vi "OpenVIFile.vi"(7 "error in (no error)":errorcluster, 8 "Pdf file path":path) -> (1 "error out":errorcluster)   [LabVIEW 2015]
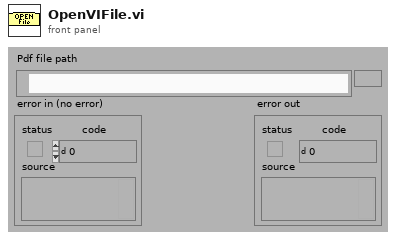
[diagram p1: front panel]
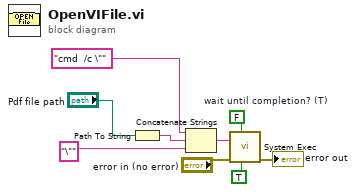
[diagram p0: block diagram]
diagram:
  w9 = FALSE  # wait until completion? (T)
  n1 = Path To String(path="Pdf file path") -> (string=w4:string)
  n2 = Concatenate Strings("cmd  /c \"", w4, "\"") -> (w6:string)
  n3 = call <vilib>:"System Exec.vi"("run minimized? (F)"=TRUE, "wait until completion? (T)"=w9, "error in (no error)"="error in (no error)", "command line"=w6) -> ("error out"=→"error out":errorcluster)  [unwired: 2 in, 5 out]
